vi "TempConversion.vi"() -> ()   [LabVIEW 2018]
uses:
  <vilib>/express/express arith-compare/Formula/XNode/ExpressFormulaBlockNode.xnode
panel:
  in  "Conversion Selector":bool
  out "?":string="Celsius"
  out "?":string
  in  "Stop Button":bool
  in  "Calculate":bool
  out "Output Temperature":dbl=32.0
  in  "Input Temperature":dbl
  # "F -> C"
  # "C -> F"
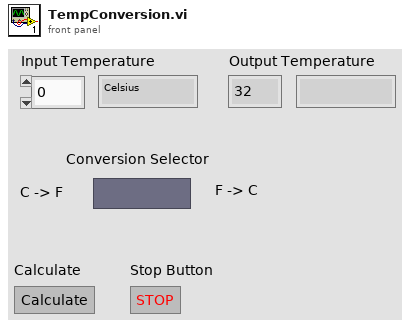
[diagram p1: front panel]
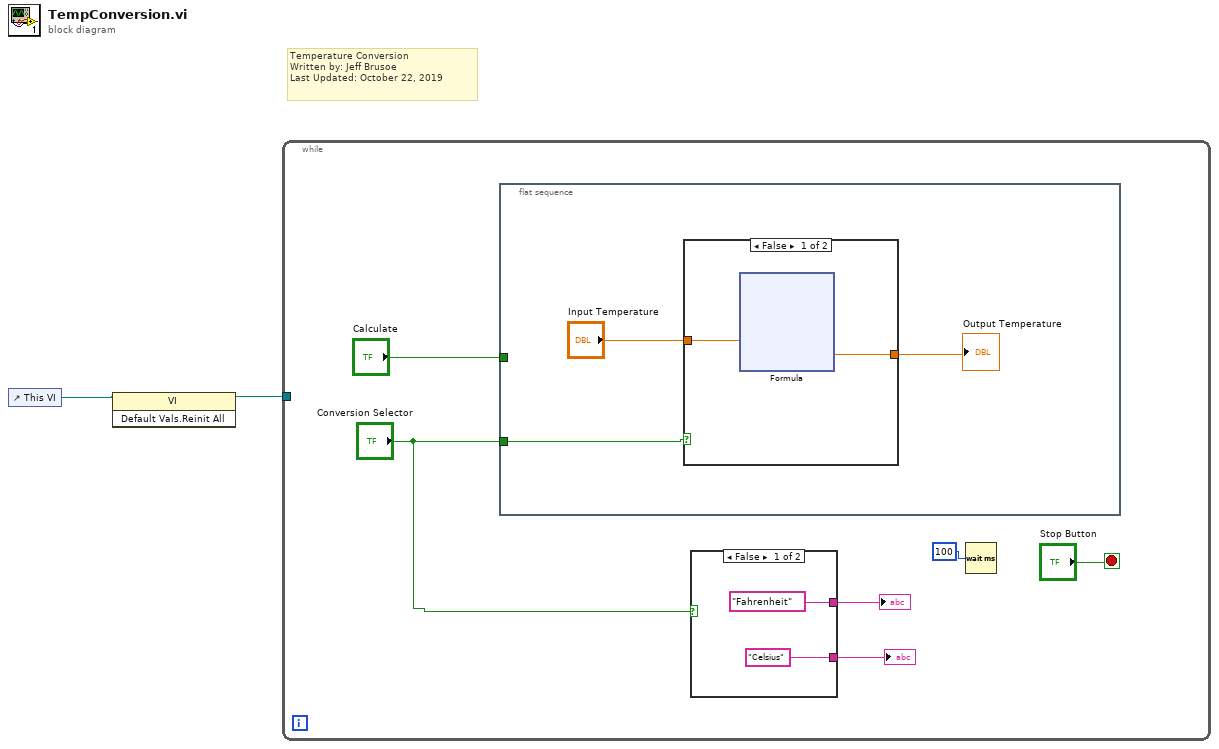
[diagram p0: block diagram]
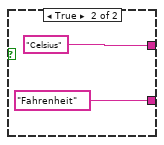
[diagram p2: hidden frame]
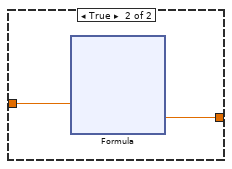
[diagram p3: hidden frame]
diagram:
  # "Temperature Conversion\nWritten by: Jeff Brusoe\nLast Updated: October 22, 2019"
  n1 = control-ref of="This VI"() -> (w2:refnum<vi>)
  n2 = invoke class="VI" method="Default Vals.Reinit All"(reference=w2) -> (reference out=w1:refnum<vi>)  [unwired: 2 in, 2 out]
  n3 = while {
    tunnel: w1 -> [_]
    stop <- "Stop Button" stop-if-true
    n4 = flat-sequence {
      tunnel: "Conversion Selector" -> [w13]
      tunnel: "Calculate" -> [_]
      frame #0 {
        n5 = case shown="False" w13 {
          tunnel: "Input Temperature" -> [w17 w27]
          tunnel: [w16 w26] -> w14
          frame False {
            n6 = xnode "Formula"("Temp"=w17) -> ("Result"=w16:dbl)  [unwired: 1 in, 1 out]
          }
          frame True {
            n7 = xnode "Formula"("Temp"=w27) -> ("Result"=w26:dbl)  [unwired: 1 in, 1 out]
          }
        }
        "Output Temperature" <- w14
      }
    }
    n8 = case shown="False" "Conversion Selector" {
      tunnel: ["Celsius" "Fahrenheit"] -> w6
      tunnel: ["Fahrenheit" "Celsius"] -> w5
      frame False {
      }
      frame True {
      }
    }
    "?" <- w6
    "?" <- w5
    n9 = Wait (ms)(milliseconds to wait=u32 100) -> ()  [unwired: 1 out]
  }
